vi "Open Sysdef and Modify Existing Custom Device.vi"() -> ()   [LabVIEW 2010]
uses:
  Read RefMem PtByPt System Definition API.lvlibp/API/Channel Config.ctl
  Read RefMem PtByPt System Definition API.lvlibp/Custom Device/Controls/Data Channel Type.ctl
  Read RefMem PtByPt System Definition API.lvlibp
  Read RefMem PtByPt System Definition API.lvlibp/Custom Device/RefMem PtByPt Custom Device.lvlib
panel:
  in  "New CPU Assignment":i32=1
  in  "New VISA Name":string="Blah"
  in  "Data Folder to Add":string="MyOtherFolder"
  in  "Data Channel Config":T1[](array[typedef])=[{"Units"="blah", "Default Value"=0.0, "Address"=0, "Description"="", "Type"=enum."Read"}, {"Units"="blah", "Default Value"=1.0, "Address"=8, "Description"="", "Type"=enum."Read"}] {"Address" format="%.0x"}
  in  "Data Channels to Add to Folder":string[](array[string])=["MyChan1", "MyChan2"]
  in  "Sysdef File to open":path
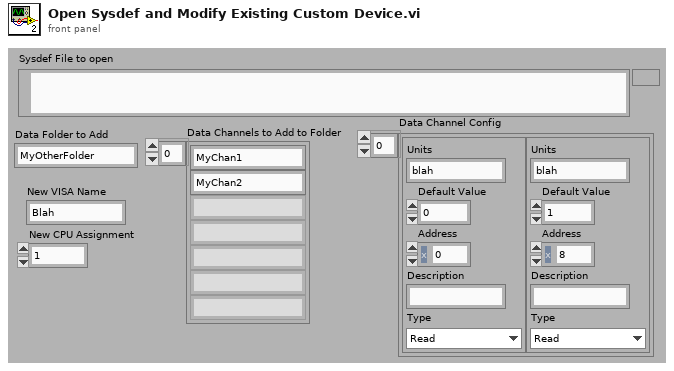
[diagram p1: front panel]
types:
  T1 = typedef "Read RefMem PtByPt System Definition API.lvlibp/Channel Config.ctl" = cluster{"Units":string, "Default Value":dbl, "Address":u32, "Description":string, "Type":T2}
  T2 = typedef "Read RefMem PtByPt System Definition API.lvlibp/RefMem PtByPt Custom Device.lvlib/Data Channel Type.ctl" = enum16{"Read", "Write"}
  T3 = typedef "SysDefRefs.ctl" = cluster{"SysDef Ref":refnum<k24>, "Root Node":refnum<k24>, "Targets Section":refnum<k24>, "Target List":refnum<k24>[], "CD Section":refnum<k24>, "CustomDeviceList":refnum<k24>[]}
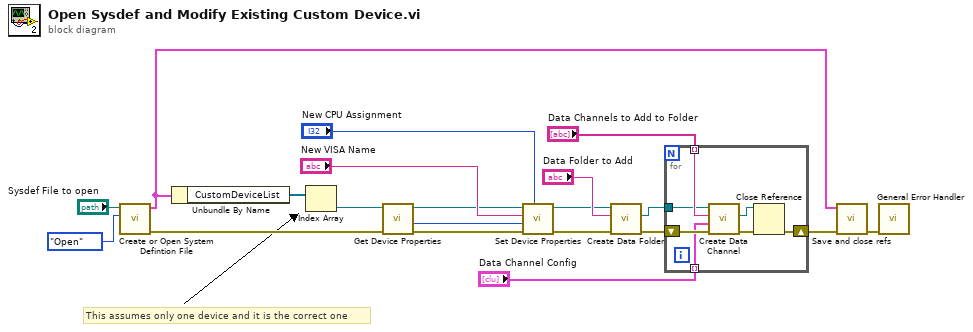
[diagram p0: block diagram]
diagram:
  # "This assumes only one device and it is the correct one"
  n1 = call "Create or Open System Defintion File.vi"("File Action"=enum16{"Open", "Create"}."Open", "Sysdef File"="Sysdef File to open") -> ("error out"=w6:errorcluster, "SysDef Refs"=w18:T3)  [unwired: 8 in]
  n2 = Unbundle By Name(w18) -> ("CustomDeviceList"=w16:refnum<k24>[])
  n3 = Index Array(array=w16) -> (element=w5:refnum<k24>)  [unwired: 1 in]
  n4 = call "Get Device Properties.vi"("error in (no error)"=w6, "Custom Device"=w5) -> ("error out"=w4:errorcluster, "Decimation"=w3:i32, "Custom Device Duplicate"=w2:refnum<k24>)  [unwired: 5 in, 2 out]
  n5 = call "Set Device Properties.vi"("CPU Assignment (-2)"="New CPU Assignment", "error in (no error)"=w4, "Decimation (1)"=w3, "VISA Name"="New VISA Name", "Custom Device"=w2) -> ("error out"=w9:errorcluster, "Custom Device Duplicate"=w8:refnum<k24>)  [unwired: 5 in]
  n6 = call "Create Data Folder.vi"("error in (no error)"=w9, "Name"="Data Folder to Add", "Parent Section"=w8) -> ("error out"=w15:errorcluster, "New Section"=w14:refnum<k24>)  [unwired: 5 in, 2 out]
  n7 = for {
    shift-right: [w23] -> w10
    shift-left: w15 -> [w27]
    tunnel: "Data Channels to Add to Folder" -> [w26] mode=indexing
    tunnel: w14 -> [w25]
    tunnel: "Data Channel Config" -> [w24] mode=indexing
    n8 = call "Create Data Channel.vi"("error in (no error)"=w27, "Channel"=w24, "Name"=w26, "Parent Section"=w25) -> ("error out"=w22:errorcluster, "New Data Channel"=w21:refnum<k24>)  [unwired: 3 in, 3 out]
    n9 = Close Reference(reference=w21, error in (no error)=w22) -> (error out=w23:errorcluster)
  }
  n10 = call "Save and close refs.vi"("error in (no error)"=w10, "SysDef Refs in"=w18) -> ("error out"=w19:errorcluster)  [unwired: 9 in]
  n11 = call <vilib>:"General Error Handler.vi"("error in (no error)"=w19) -> ()  [unwired: 10 in, 5 out]
